vi "input.vi"(2 "位数(2)":i32=2, 3 "in":dbl=1.2345) -> (0 "out":dbl format="%.6f", 1 "值改变?":bool)   [LabVIEW 2018]
panel:
  in  "ESC":bool
  in  "C":bool
  in  "字符串":string
  in  ".":bool
  in  "0":bool
  in  "-":bool
  in  "bk":bool
  in  "en":bool
  in  "3":bool
  in  "2":bool
  in  "1":bool
  in  "6":bool
  in  "5":bool
  in  "4":bool
  in  "9":bool
  in  "8":bool
  in  "7":bool
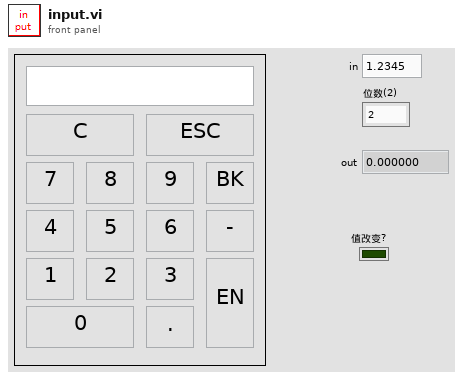
[diagram p1: front panel]
types:
  T1 = enum8{"Enabled", "Disabled", "Disabled and Grayed Out"}
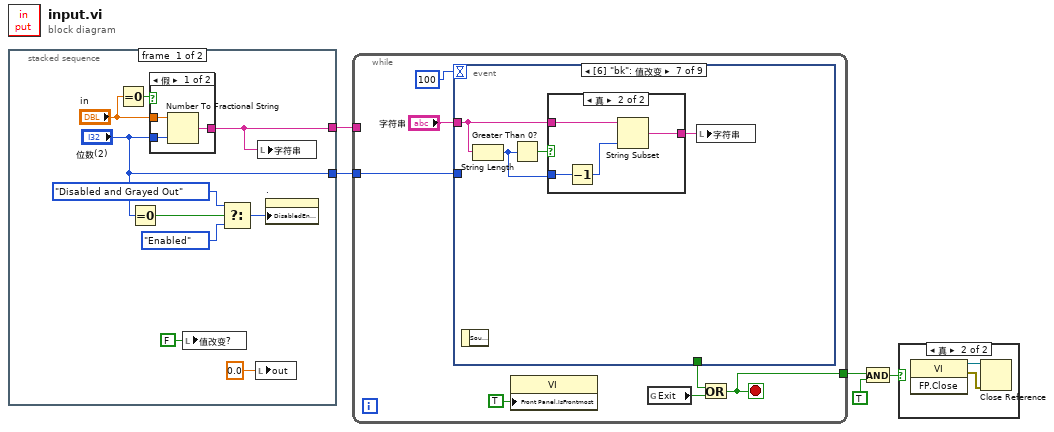
[diagram p0: block diagram]
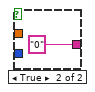
[diagram p2: hidden frame]
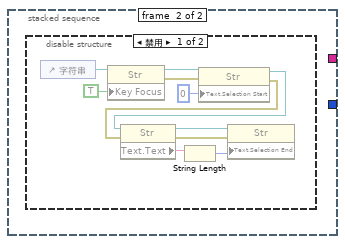
[diagram p3: hidden frame]
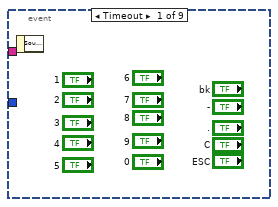
[diagram p6: hidden frame]
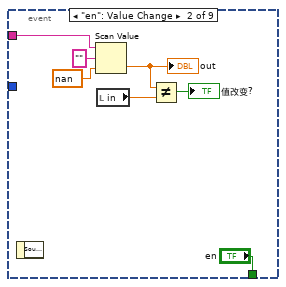
[diagram p7: hidden frame]
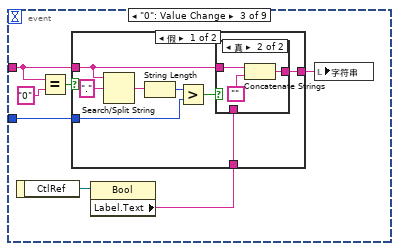
[diagram p8: hidden frame]
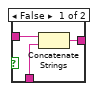
[diagram p9: hidden frame]
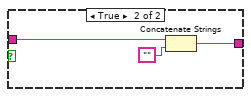
[diagram p10: hidden frame]
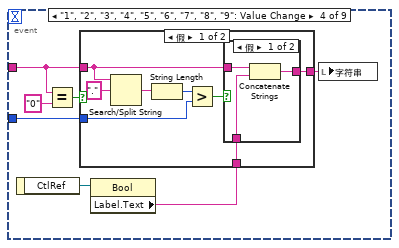
[diagram p11: hidden frame]
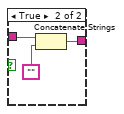
[diagram p12: hidden frame]
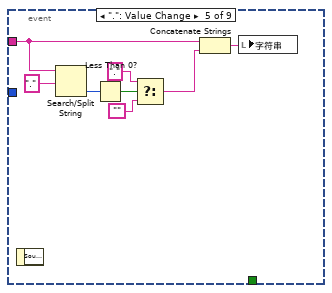
[diagram p14: hidden frame]
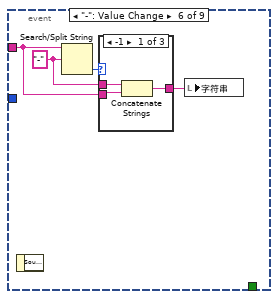
[diagram p15: hidden frame]
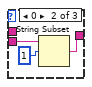
[diagram p16: hidden frame]
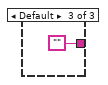
[diagram p17: hidden frame]
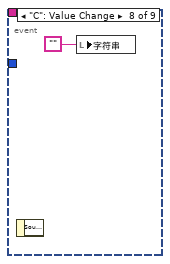
[diagram p19: hidden frame]
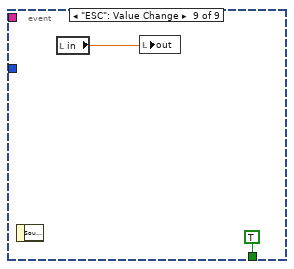
[diagram p20: hidden frame]
diagram:
  n1 = stacked-sequence {
    tunnel: [w15 _] -> w5
    tunnel: ["位数(2)" _] -> w1
    frame #0 {
      n2 = Equal To 0?(x="in") -> (x = 0?=w13:bool)
      n3 = Equal To 0?(x="位数(2)") -> (x = 0?=w9:bool)
      n4 = case shown="假" w13 {
        tunnel: "in" -> [w18 _]
        tunnel: [w17 "0"] -> w15
        tunnel: "位数(2)" -> [w16 _]
        frame False {
          n5 = Number To Fractional String(number=w18, precision (6)=w16) -> (F-format string=w17:string)  [unwired: 2 in]
        }
        frame True {
        }
      }
      n6 = local write "值改变?"(FALSE ("值改变")) -> ()
      n7 = Select(t=T1."Disabled and Grayed Out" ("禁用"), s=w9, f=T1."Enabled" ("禁用")) -> (s? t:f=w8:T1)
      n8 = local write "out"(0.0) -> ()
      n9 = local write "字符串"(w15) -> ()
      n10 = property on="." class="Bool"("DisabledEnum"=w8) -> ()  [unwired: 2 in, 2 out]
    }
    frame #1 {
      n11 = disable-structure shown="禁用" {
        frame Disabled {
          n12 = control-ref of="字符串"() -> (w28:refnum<vi>)
          n13 = property class="Str"(reference=w28, "Key Focus"=TRUE ("键选中")) -> (reference out=w25:refnum<vi>, error out=w24:errorcluster)  [unwired: 1 in]
          n14 = property class="Str"(reference=w25, error in=w24, "Text.Selection Start"=u32 0 ("文本.选择区域:起始")) -> (reference out=w21:refnum<vi>, error out=w22:errorcluster)
          n15 = property class="Str"(reference=w21, error in=w22) -> (reference out=w29:refnum<vi>, error out=w20:errorcluster, "Text.Text"=w30:string)
          n16 = String Length(string=w30) -> (length=w26:i32)
          n17 = property class="Str"(reference=w29, error in=w20, "Text.Selection End"=w26) -> ()  [unwired: 2 out]
        }
        frame Enabled {
        }
      }
    }
  }
  n18 = while {
    tunnel: [w34] -> w4
    tunnel: w5 -> [_]
    tunnel: w1 -> [w31]
    stop <- w34 stop-if-true
    n19 = event shown="[6] \"bk\": 值改变" {
      selector: _ -> [_ _ _ _ _ _ _ _ _]
      dyn-events: _ -> [_ _ _ _ _ _ _ _ _]
      timeout: 100 -> [_ _ _ _ _ _ _ _ _]
      tunnel: [_ "en" _ _ _ _ _ _ TRUE ("en")] -> w33
      tunnel: "字符串" -> [_ w43 w50 w70 w97 w100 w111 _ _]
      tunnel: w31 -> [_ _ w46 w69 _ _ _ _ _]
      event Timeout {
        n20 = event-data() -> ()  [unwired: 1 in, 1 out]
      }
      event "en": Value Change {
        n21 = event-data() -> ()  [unwired: 1 in, 1 out]
        n22 = Scan Value(string=w43, format string="" ("格式字符串"), default (0 dbl)=nan ("默认(0 dbl)")) -> (value=w41:dbl)  [unwired: 1 out]
        "out" <- w41
        n23 = local read "in"() -> (w40:dbl)
        n24 = Not Equal?(x=w41, y=w40) -> (x != y?=→"值改变?":bool)
      }
      event "0": Value Change {
        n25 = event-data() -> ("CtlRef"=w47:refnum<vi>)  [unwired: 1 in]
        n26 = Equal?(x=w50, y="0") -> (x = y?=w48:bool)
        n27 = property class="Bool"(reference=w47) -> ("Label.Text"=w45:string)  [unwired: 1 in, 2 out]
        n28 = case shown="假" w48 {
          tunnel: w50 -> [w53 w68]
          tunnel: [w54 w67] -> w49
          tunnel: w46 -> [w56 _]
          tunnel: w45 -> [w52 _]
          frame False {
            n29 = Search/Split String(string=w53, search string/char (-)="." ("搜索字符串/字符(-)")) -> (match + rest of string=w58:string)  [unwired: 1 in, 2 out]
            n30 = String Length(string=w58) -> (length=w57:i32)
            n31 = Greater?(x=w57, y=w56) -> (0:w55:bool)
            n32 = case shown="真" w55 {
              tunnel: [w62 w64] -> w54
              tunnel: w53 -> [w61 w63]
              tunnel: w52 -> [w60 _]
              frame False {
                n33 = Concatenate Strings(w61, w60) -> (w62:string)
              }
              frame True {
                n34 = Concatenate Strings(w63, "") -> (w64:string)
              }
            }
          }
          frame True {
            n35 = Concatenate Strings(w68, "") -> (w67:string)
          }
        }
        n36 = local write "字符串"(w49) -> ()
      }
      event "1", "2", "3", "4", "5", "6", "7", "8", "9": Value Change {
        n37 = event-data() -> ("CtlRef"=w75:refnum<vi>)  [unwired: 1 in]
        n38 = Equal?(x=w70, y="0") -> (x = y?=w73:bool)
        n39 = property class="Bool"(reference=w75) -> ("Label.Text"=w72:string)  [unwired: 1 in, 2 out]
        n40 = case shown="假" w73 {
          tunnel: w72 -> [w76 w90]
          tunnel: [w83 w90] -> w71
          tunnel: w70 -> [w82 _]
          tunnel: w69 -> [w78 _]
          frame False {
            n41 = Search/Split String(string=w82, search string/char (-)="." ("搜索字符串/字符(-)")) -> (match + rest of string=w80:string)  [unwired: 1 in, 2 out]
            n42 = String Length(string=w80) -> (length=w79:i32)
            n43 = Greater?(x=w79, y=w78) -> (0:w77:bool)
            n44 = case shown="假" w77 {
              tunnel: [w86 w89] -> w83
              tunnel: w82 -> [w85 w88]
              tunnel: w76 -> [w84 _]
              frame False {
                n45 = Concatenate Strings(w85, w84) -> (w86:string)
              }
              frame True {
                n46 = Concatenate Strings(w88, "") -> (w89:string)
              }
            }
          }
          frame True {
          }
        }
        n47 = local write "字符串"(w71) -> ()
      }
      event ".": Value Change {
        n48 = event-data() -> ()  [unwired: 1 in, 1 out]
        n49 = Search/Split String(string=w97, search string/char (-)=".") -> (offset of match=w95:i32)  [unwired: 1 in, 2 out]
        n50 = Less Than 0?(x=w95) -> (x < 0?=w94:bool)
        n51 = Select(t=".", s=w94, f="") -> (s? t:f=w92:string)
        n52 = Concatenate Strings(w97, w92) -> (w98:string)
        n53 = local write "字符串"(w98) -> ()
      }
      event "-": Value Change {
        w101 = "-" ("搜索字符串/字符(-)")
        n54 = event-data() -> ()  [unwired: 1 in, 1 out]
        n55 = Search/Split String(string=w100, search string/char (-)=w101) -> (offset of match=w102:i32)  [unwired: 1 in, 2 out]
        n56 = case shown="-1" w102 {
          tunnel: w101 -> [w105 _ _]
          tunnel: w100 -> [w104 w108 _]
          tunnel: [w103 w106 ""] -> w99
          frame -1 {
            n57 = Concatenate Strings(w105, w104) -> (w103:string)
          }
          frame 0 {
            n58 = String Subset(string=w108, offset (0)=1 ("偏移量(0)")) -> (substring=w106:string)  [unwired: 1 in]
          }
          frame Default {
          }
        }
        n59 = local write "字符串"(w99) -> ()
      }
      event "bk": Value Change {
        n60 = event-data() -> ()  [unwired: 1 in, 1 out]
        n61 = String Length(string=w111) -> (length=w110:i32)
        n62 = Greater Than 0?(x=w110) -> (x > 0?=w112:bool)
        n63 = case shown="真" w112 {
          tunnel: [w114 w118] -> w113
          tunnel: w111 -> [w114 w117]
          tunnel: w110 -> [_ w116]
          frame False {
          }
          frame True {
            n64 = Decrement(x=w116) -> (x-1=w115:i32)
            n65 = String Subset(string=w117, length (rest)=w115) -> (substring=w118:string)  [unwired: 1 in]
          }
        }
        n66 = local write "字符串"(w113) -> ()
      }
      event "C": Value Change {
        n67 = event-data() -> ()  [unwired: 1 in, 1 out]
        n68 = local write "字符串"("") -> ()
      }
      event "ESC": Value Change {
        n69 = event-data() -> ()  [unwired: 1 in, 1 out]
        n70 = local read "in"() -> (w121:dbl)
        n71 = local write "out"(w121) -> ()
      }
    }
    n72 = property class="VI"("Front Panel.IsFrontmost"=TRUE) -> ()  [unwired: 2 in, 2 out]
    n73 = global read "全局 1.vi" "Exit"() -> (w32:bool)
    n74 = Or(x=w33, y=w32) -> (x .or. y?=w34:bool)
  }
  n75 = And(x=w4, y=TRUE) -> (x .and. y?=w3:bool)
  n76 = case shown="真" w3 {
    frame False {
    }
    frame True {
      n77 = invoke class="VI" method="FP.Close"() -> (reference out=w122:refnum<vi>, error out=w123:errorcluster)  [unwired: 3 in, 1 out]
      n78 = Close Reference(reference=w122, error in (no error)=w123) -> ()  [unwired: 1 out]
    }
  }
